vi "CloseDevice.vi"(8 "error in (no error)":errorcluster, 11 "Device Index":i32) -> (0 "error out":errorcluster)   [LabVIEW 2019, in "TopasDriver.lvlib"]
uses:
  TopasDriver.lvlib
  TopasAPI.dll
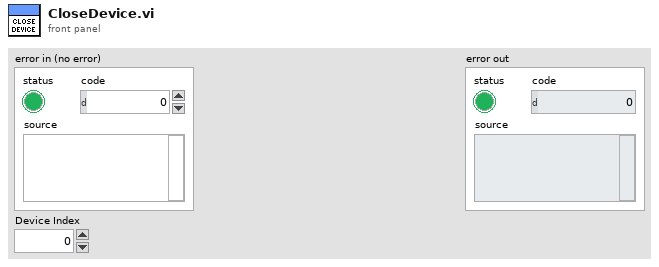
[diagram p1: front panel]
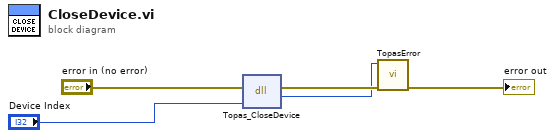
[diagram p0: block diagram]
diagram:
  n1 = dll-call lib="G:/LabVIEW/Topas-LabVIEW-Driver/Libraries/TopasAPI.dll" fn="Topas_CloseDevice"(error in="error in (no error)", "index"="Device Index") -> (error out=w3:errorcluster, "return type"=w1:u64)  [unwired: 3 in, 1 out]
  n2 = call "TopasError.vi"("error in"=w3, "Error Code"=w1) -> ("error out"=→"error out":errorcluster)  [unwired: 9 in]
